vi "Subsys02_Main.vi"() -> ()   [LabVIEW 2019]
uses:
  Subsys02_Global.vi
panel:
  out "V02":dbl
  out "V01":dbl
  out "status":u32(colorbox)
  in  "stop":bool
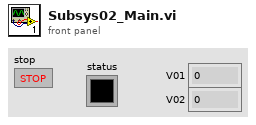
[diagram p1: front panel]
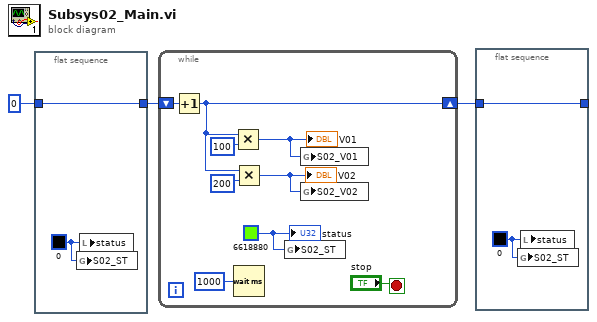
[diagram p0: block diagram]
diagram:
  n1 = flat-sequence {
    tunnel: 0 -> [w4]
    tunnel: [w4] -> w2
    frame #0 {
      w5 = u32 0 ("status")
      n2 = global write "Subsys02_Global.vi" "S02_ST"(w5) -> ()
      n3 = local write "status"(w5) -> ()
    }
  }
  n4 = while {
    shift-right: [w9] -> w1
    shift-left: w2 -> [w14]
    stop <- "stop" stop-if-true
    w10 = u32 6618880 ("alarm_status")
    n5 = Increment(x=w14) -> (x+1=w9:i32)
    n6 = Multiply(x=w9, y=100) -> (x*y=w6:i32)
    "V01" <- w6
    n7 = Multiply(x=w9, y=200) -> (x*y=w7:i32)
    "V02" <- w7
    n8 = Wait (ms)(milliseconds to wait=u32 1000) -> ()  [unwired: 1 out]
    n9 = global write "Subsys02_Global.vi" "S02_ST"(w10) -> ()
    n10 = global write "Subsys02_Global.vi" "S02_V01"(w6) -> ()
    n11 = global write "Subsys02_Global.vi" "S02_V02"(w7) -> ()
    "status" <- w10
  }
  n12 = flat-sequence {
    tunnel: w1 -> [w15]
    tunnel: [w15] -> _
    frame #0 {
      w16 = u32 0 ("status")
      n13 = global write "Subsys02_Global.vi" "S02_ST"(w16) -> ()
      n14 = local write "status"(w16) -> ()
    }
  }
